vi "Set Time Zone.vi"(0 "GMaps API in":refnum<class "GMaps API.lvclass">, 1 "Latitude":string, 2 "Longitude":string, 5 "error in (no error)":errorcluster) -> (14 "GMaps API out":refnum<class "GMaps API.lvclass">, 19 "error out":errorcluster)   [LabVIEW 2016, in "GMaps API.lvclass"]
doc: "Sets offset data for location on the surface of the earth."
uses:
  GMaps API.lvclass
  GMaps API.lvclass/GMaps API.ctl
  <vilib>/regexp/Match Regular Expression.xnode
  <vilib>/httpClient/LabVIEWHTTPClient.lvlib
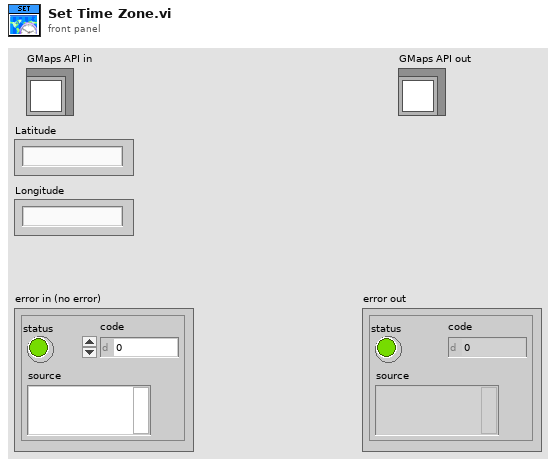
[diagram p1: front panel]
types:
  T1 = typedef "LVDateTimeRec.ctl" = cluster{"fractional second":dbl, "second":i32, "minute":i32, "hour":i32, "day of month":i32, "month":i32, "year":i32, "day of week":i32, "day of year":i32, "DST":i32}
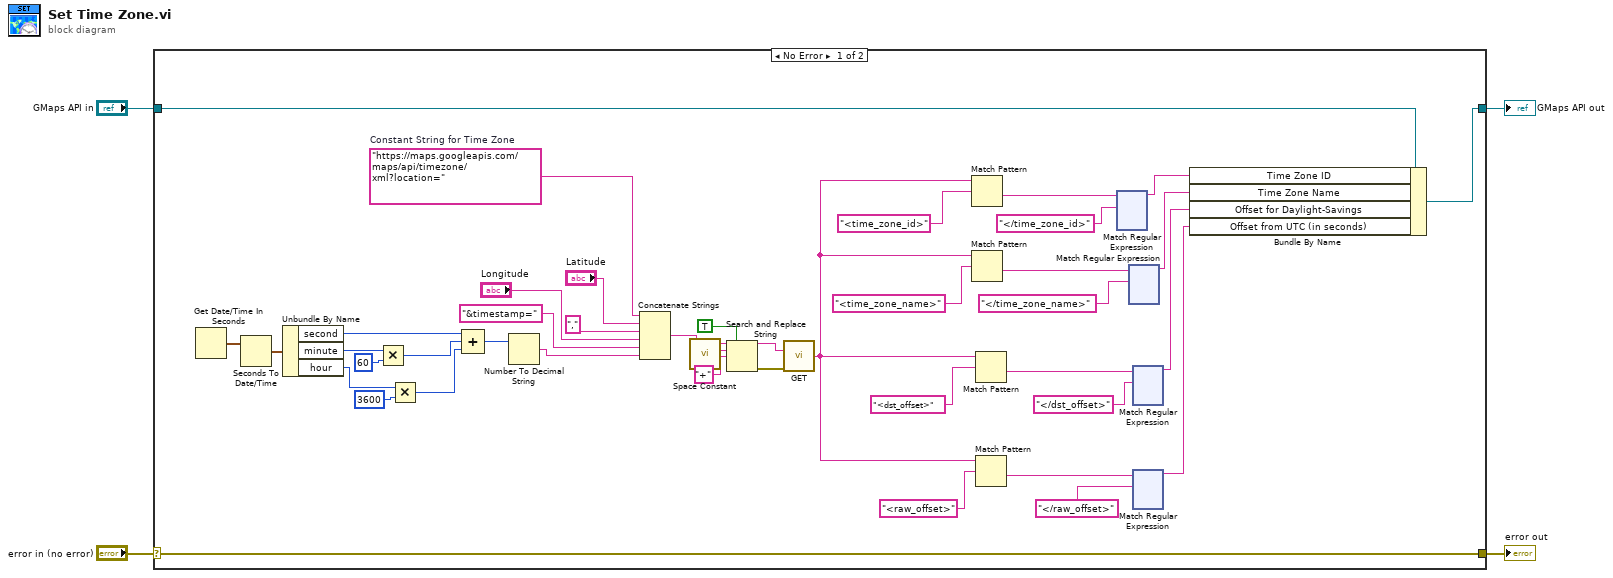
[diagram p0: block diagram]
diagram:
  n1 = case shown="No Error" "error in (no error)" {
    selector: "error in (no error)" -> [w46 w504]
    tunnel: [w46 w504] -> w3
    tunnel: [w5 w503] -> w1
    tunnel: "GMaps API in" -> [w10 w503]
    frame No Error {
      w26 = "https://maps.googleapis.com/maps/api/timezone/xml?location="  # Constant String for Time Zone
      n2 = Get Date/Time In Seconds() -> (seconds since 1Jan1904=w45:timestamp)
      n3 = Seconds To Date/Time(time stamp (now)=w45) -> (date time rec=w44:T1)  [unwired: 1 in]
      n4 = Unbundle By Name(w44) -> ("second"=w39:i32, "minute"=w43:i32, "hour"=w40:i32)
      n5 = Multiply(x=w43, y=60) -> (x*y=w38:i32)
      n6 = Multiply(x=w40, y=3600) -> (x*y=w37:i32)
      n7 = Compound Arithmetic op=ADD(w39, w38, w37) -> (w36:i32)
      n8 = Number To Decimal String(number=w36) -> (decimal integer string=w23:string)  [unwired: 1 in]
      n9 = Concatenate Strings(w26, "Latitude", ",", "Longitude", "&timestamp=", w23) -> (w22:string)
      n10 = call <vilib>:"Space Constant.vi"() -> ("String"=w32:string)
      n11 = Search and Replace String(replace all?=TRUE ("replace all? (F)"), input string=w22, search string=w32, replace string="+" ("replace string (\"\")")) -> (result string=w21:string, error out=w34:errorcluster)  [unwired: 4 in, 2 out]
      n12 = call <vilib>:"GET.vi"("url"=w21, "error in (no error)"=w34) -> ("body"=w13:string)  [unwired: 10 in, 3 out]
      n13 = Match Pattern(string=w13, regular expression="<time_zone_id>" ("Directly After Latitude info")) -> (after substring=w28:string)  [unwired: 4 out]
      n14 = Match Pattern(string=w13, regular expression="<time_zone_name>" ("Directly Before Latitude info")) -> (after substring=w27:string)  [unwired: 4 out]
      n15 = Match Pattern(string=w13, regular expression="<dst_offset>" ("Directly Before Latitude info")) -> (after substring=w19:string)  [unwired: 4 out]
      n16 = Match Pattern(string=w13, regular expression="<raw_offset>" ("Directly Before Latitude info")) -> (after substring=w14:string)  [unwired: 4 out]
      n17 = xnode "Match Regular Expression"("input string"=w28, "regular expression"="</time_zone_id>") -> ("before match"=w9:string)  [unwired: 4 in, 4 out]
      n18 = xnode "Match Regular Expression"("input string"=w27, "regular expression"="</time_zone_name>" ("Directly After Latitude info")) -> ("before match"=w8:string)  [unwired: 4 in, 4 out]
      n19 = xnode "Match Regular Expression"("input string"=w19, "regular expression"="</dst_offset>" ("Directly After Latitude info")) -> ("before match"=w7:string)  [unwired: 4 in, 4 out]
      n20 = xnode "Match Regular Expression"("input string"=w14, "regular expression"="</raw_offset>" ("Directly After Latitude info")) -> ("before match"=w6:string)  [unwired: 4 in, 4 out]
      n21 = Bundle By Name(cluster=w10, "Time Zone ID"=w9, "Time Zone Name"=w8, "Offset for Daylight-Savings"=w7, "Offset from UTC (in seconds)"=w6) -> (w5:refnum<class "GMaps API.lvclass">)
    }
    frame Error {
    }
  }
  "error out" <- w3
  "GMaps API out" <- w1
